vi "cRIO Main.vi"() -> ()   [LabVIEW 2013]
doc: "This example runs a background service that initializes and interacts with the Tag Bus Data framework. The service is designed to run continuously so that the framework can be reinitialized with a new configuration without rebooting the target. This can save time when iterating on a configuration.\n\nThe example includes a collection of VIs for sending and receiving messages from the engine service."
uses:
  TBD Message Service/SubVIs/command commands to rtexe process.ctl
  TBD Message Service/SubVIs/engine status data.ctl
  <vilib>/NI/Module Execution Interface/Engine Runtime/Execution States.ctl
  <vilib>/NI/Module Execution Interface/Engine Runtime/Fault.ctl
  <vilib>/NI/Tag Bus Module Framework/runtime/error classification.ctl
  TBD Message Service/SubVIs/queue name.ctl
  <vilib>/NI/Current Value Table/DataTypes/Double_Read.vi
  <vilib>/NI/Current Value Table/Type to Enum.vi
  <vilib>/NI/Current Value Table/DataTypes/Double_Type To Enum.vi
  <vilib>/NI/AMC/Read Termination Message.vi
  TBD Message Service/SubVIs/command to string.vi
  TBD Message Service/SubVIs/string to commands.vi
  <vilib>/NI/AMC/Create Single Message.vi
  <vilib>/NI/Current Value Table/FGVs/CVT Globals.vi
  <vilib>/NI/Current Value Table/FGVs/Tag Memory.vi
  <vilib>/NI/Current Value Table/Memory Block.vi
  <vilib>/NI/Current Value Table/DataTypes/Double_Memory Block.vi
  <vilib>/NI/AMC/Globals.vi
  TBD Message Service/TBD message service.lvlib
  <vilib>/NI/AMC/AMC.lvlib
  <vilib>/NI/Current Value Table/Current Value Table.lvlib
  <vilib>/NI/Module Execution Interface/Engine Runtime/Engine Runtime Interface.lvclass
  <vilib>/NI/Tag Bus Module Framework/runtime/TBM module execution interface.lvclass
panel:
  in  "Exit":bool
  in  "Reload":bool
  out "timed structures load":dbl
  out "CPU load average":dbl
  out "final error":errorcluster
  out "Lamp PWM":cluster{"Value":dbl, "Value":dbl}(graph)
  out "Temperature":cluster{"Value":dbl, "Value":dbl}(graph)
  out "system error":errorcluster
  out "engine statuses":T1[](array[typedef])
  out "command error":errorcluster
  out "commands":T5
  out "engine loaded":string
  out "load error":errorcluster
  out "Invalid Message":string
  in  "config. file path":path=path "/home/lvuser/natinst/bin/FullSystem.pcfg"
  # "Status Information"
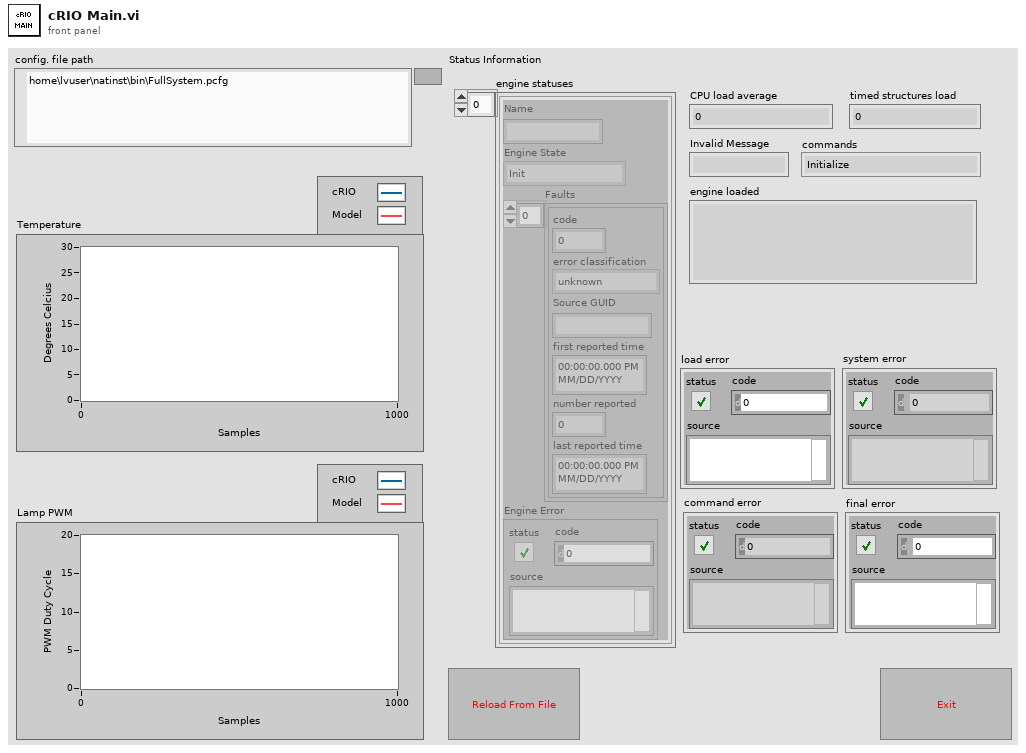
[diagram p1: front panel]
types:
  T1 = typedef "TBD message service.lvlib/engine status data.ctl" = cluster{"Name":string, "Engine State":T2, "Faults":T3[], "Engine Error":errorcluster}
  T2 = typedef "Engine Runtime Interface.lvclass/Execution States.ctl" = enum16{"Init", "Pre-Operational", "Safe-Operational", "Operational", "Stopped"}
  T3 = typedef "Engine Runtime Interface.lvclass/Fault.ctl" = cluster{"code":i32, "error classification":T4, "Source GUID":string, "first reported time":timestamp, "number reported":u32, "last reported time":timestamp}
  T4 = typedef "TBM module execution interface.lvclass/error classification.ctl" = enum16{"unknown", "none", "trivial", "recoverable", "critical"}
  T5 = typedef "TBD message service.lvlib/command commands to rtexe process.ctl" = enum16{"Initialize", "Add Search Paths", "Load from File", "Unload File", "Open All Engines", "Open Single Engine", "Initialize All Engines", "Initialize Single Engine", "Start All", "Start Single", "Pause All", "Pause Single", "Stop All", "Stop Single", "Close All", "Close Single", "Set Safe State All", "Set Safe State Single", "Get Status", "Exit", "Error", "Load Bitfile", "Unload Bitfile", "Clear Faults Single", "Clear Faults All"}
  T6 = typedef "TBD message service.lvlib/queue name.ctl" = enum16{"TOrtmainexec", "FROMrtmainexec"}
  T7 = typedef "AMC.lvlib/Message Queue.ctl" = refnum<queue>
  T8 = typedef "TBD message service.lvlib/common reponses to network process.ctl" = enum16{"System Error", "Load Report", "Action Response", "Engine Status"}
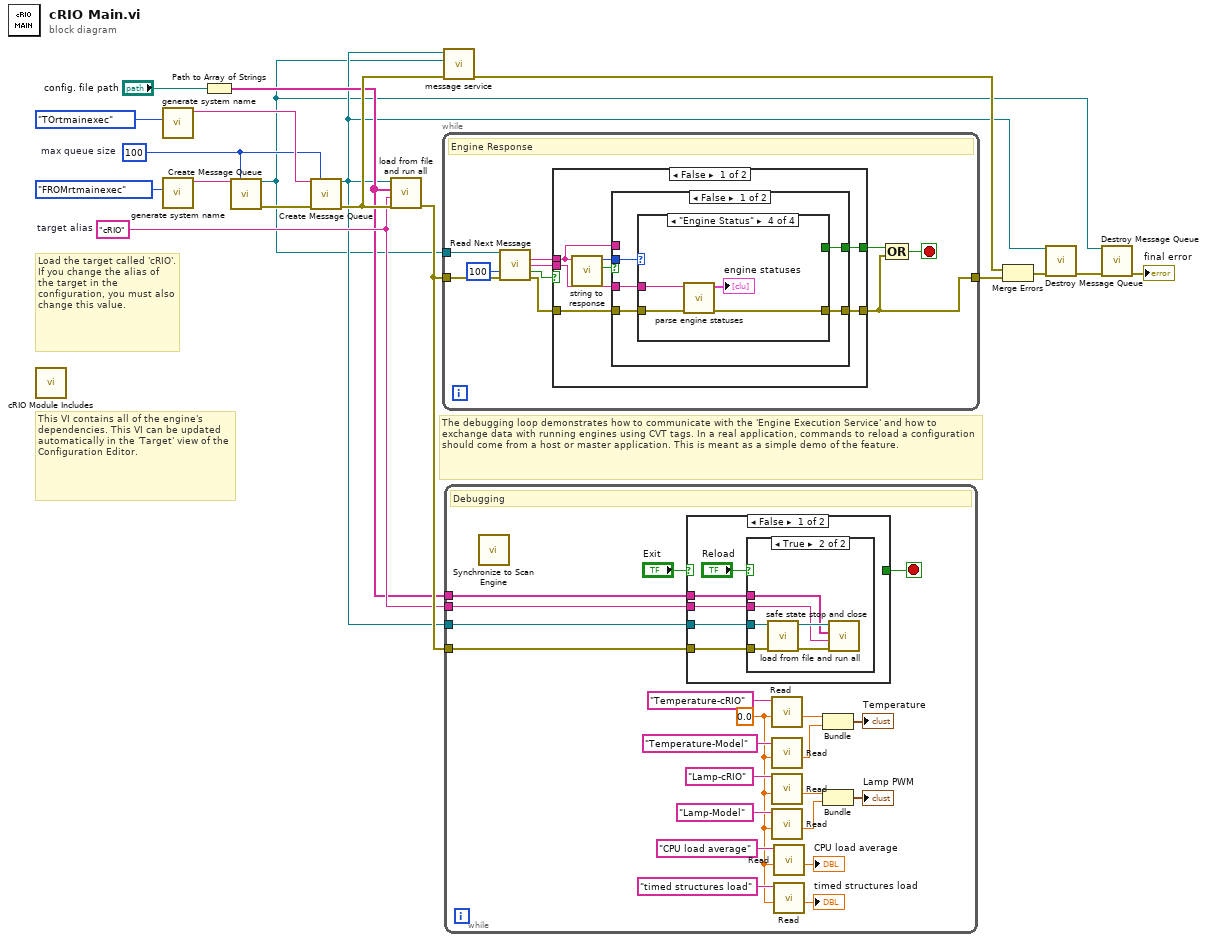
[diagram p0: block diagram]
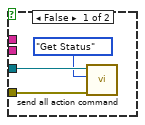
[diagram p2: hidden frame]
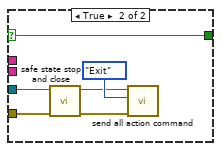
[diagram p3: hidden frame]
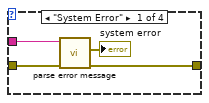
[diagram p4: hidden frame]
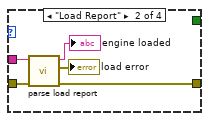
[diagram p5: hidden frame]
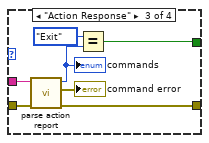
[diagram p6: hidden frame]
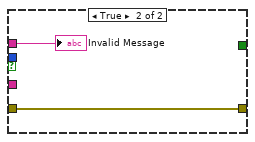
[diagram p7: hidden frame]
diagram:
  w12 = 100  # max queue size
  w9 = "cRIO"  # target alias
  # "This VI contains all of the engine's dependencies. This VI can be updated automatically in the 'Target' view of the Configuration Editor."
  # "Load the target called 'cRIO'. If you change the alias of the target in the configuration, you must also change this value."
  # "The debugging loop demonstrates how to communicate with the 'Engine Execution Service' and how to exchange data with running engines using CVT tags. In a real application, commands to reload a configuration should come from a host or master application. This is meant as a simple demo of the feature."
  n1 = call "cRIO Module Includes.vi"() -> ()  [unwired: 12 in]
  n2 = call "generate system name.vi"("queue type"=queue_name."TOrtmainexec" ("queue")) -> ("queue name"=w16:string)  [unwired: 10 in]
  n3 = call "generate system name.vi"("queue type"=queue_name."FROMrtmainexec" ("queue")) -> ("queue name"=w18:string)  [unwired: 10 in]
  n4 = Path to Array of Strings(0:"config. file path") -> (2:w8:string[])  [unwired: 1 out]
  n5 = call <vilib>:"Create Message Queue.vi"("message queue name"=w18, "max queue size (-1, unlimited)"=w12) -> ("message queue out"=w1:T7, "error out"=w17:errorcluster)  [unwired: 12 in]
  n6 = call <vilib>:"Create Message Queue.vi"("message queue name"=w16, "max queue size (-1, unlimited)"=w12, "error in"=w17) -> ("message queue out"=w2:T7, "error out"=w11:errorcluster)  [unwired: 11 in]
  n7 = call "load from file and run all.vi"("error in"=w11, "target alias"=w9, "tokenized path"=w8, "message queue in"=w2) -> ("error out"=w10:errorcluster)  [unwired: 6 in, 1 out]
  n8 = while {
    tunnel: w1 -> [w27]
    tunnel: w10 -> [w24]
    tunnel: [w19] -> w7
    stop <- w21 stop-if-true
    # "Engine Response"
    n9 = call <vilib>:"Read Next Message.vi"("message queue in"=w27, "timeout (1 ms)"=100, "error in"=w24) -> ("message name"=w26:string, "message value"=w20:string, "timed out?"=w23:bool, "error out"=w25:errorcluster)  [unwired: 5 in, 4 out]
    n10 = case shown="False" w23 {
      tunnel: w26 -> [w29 _]
      tunnel: [w34 _] -> w22
      tunnel: w25 -> [w32 w63]
      tunnel: [w31 w63] -> w19
      tunnel: w20 -> [w30 _]
      frame False {
        n11 = call "string to response.vi"("command string"=w29) -> ("invalid"=w35:bool, "responses"=w33:T8)  [unwired: 9 in]
        n12 = case shown="False" w35 {
          tunnel: w30 -> [w39 _]
          tunnel: [w36 _] -> w34
          tunnel: w33 -> [w40 _]
          tunnel: w32 -> [w38 w62]
          tunnel: [w37 w62] -> w31
          tunnel: w29 -> [_ w61]
          frame False {
            n13 = case shown="\"Engine Status\"" w40 {
              tunnel: w39 -> [w44 w49 w56 w60]
              tunnel: w38 -> [w43 w48 w55 w59]
              tunnel: [w41 w45 w53 w58] -> w37
              tunnel: [_ _ w50 _] -> w36
              frame "System Error" {
                n14 = call "parse error message.vi"("error in"=w43, "message data"=w44) -> ("error out"=w41:errorcluster, "system error"=→"system error":errorcluster)  [unwired: 8 in]
              }
              frame "Load Report" {
                n15 = call "parse load report.vi"("error in"=w48, "message data"=w49) -> ("error out"=w45:errorcluster, "load error"=→"load error":errorcluster, "engine loaded"=→"engine loaded":string)  [unwired: 7 in]
              }
              frame "Action Response" {
                n16 = call "parse action report.vi"("error in"=w55, "message data"=w56) -> ("error out"=w53:errorcluster, "command error"=→"command error":errorcluster, "commands"=w52:T5)  [unwired: 7 in]
                "commands" <- w52
                n17 = Equal?(x=command_commands_to_rtexe_process."Exit", y=w52) -> (x = y?=w50:bool)
              }
              frame "Engine Status" {
                n18 = call "parse engine statuses.vi"("error in"=w59, "message data"=w60) -> ("error out"=w58:errorcluster, "engine statuses"=→"engine statuses":T1[])  [unwired: 8 in]
              }
            }
          }
          frame True {
            "Invalid Message" <- w61
          }
        }
      }
      frame True {
      }
    }
    n19 = Compound Arithmetic op=OR(w22, w19) -> (w21:bool)
  }
  n20 = call "message service.vi"("error in"=w11, "response queue"=w1, "command queue"=w2) -> ("error out"=w6:errorcluster)  [unwired: 8 in]
  n21 = while {
    tunnel: w10 -> [w67]
    tunnel: w2 -> [w68]
    tunnel: w8 -> [w66]
    tunnel: w9 -> [w65]
    stop <- w64 stop-if-true
    w72 = 0.0 ("Default")
    # "Debugging"
    n22 = call <vilib>:"Synchronize to Scan Engine.vi"() -> ()  [unwired: 10 in, 2 out]
    n23 = case shown="False" "Exit" {
      selector: "Exit" -> [_ w102]
      tunnel: w68 -> [w88 w104]
      tunnel: w67 -> [w87 w103]
      tunnel: w66 -> [w86 _]
      tunnel: w65 -> [w85 _]
      tunnel: [_ w102] -> w64
      frame False {
        n24 = case shown="True" "Reload" {
          tunnel: w88 -> [w92 w98]
          tunnel: w87 -> [w91 w97]
          tunnel: w86 -> [_ w94]
          tunnel: w85 -> [_ w93]
          frame False {
            n25 = call "send all action command.vi"("error in"=w91, "commands"=command_commands_to_rtexe_process."Get Status", "message queue in"=w92) -> ()  [unwired: 7 in, 2 out]
          }
          frame True {
            n26 = call "safe state stop and close.vi"("error in"=w97, "message queue in"=w98) -> ("error out"=w95:errorcluster, "message queue out"=w96:T7)  [unwired: 8 in]
            n27 = call "load from file and run all.vi"("error in"=w95, "target alias"=w93, "tokenized path"=w94, "message queue in"=w96) -> ()  [unwired: 6 in, 2 out]
          }
        }
      }
      frame True {
        n28 = call "safe state stop and close.vi"("error in"=w103, "message queue in"=w104) -> ("error out"=w99:errorcluster, "message queue out"=w100:T7)  [unwired: 8 in]
        n29 = call "send all action command.vi"("error in"=w99, "commands"=command_commands_to_rtexe_process."Exit", "message queue in"=w100) -> ()  [unwired: 7 in, 2 out]
      }
    }
    n30 = call-poly <vilib>:"Read.vi"("Default"=w72, "Tag Name"="Temperature-cRIO") -> ("Value"=w80:dbl)  [unwired: 8 in, 1 out]
    n31 = call-poly <vilib>:"Read.vi"("Default"=w72, "Tag Name"="Temperature-Model") -> ("Value"=w79:dbl)  [unwired: 8 in, 1 out]
    n32 = call-poly <vilib>:"Read.vi"("Default"=w72, "Tag Name"="Lamp-cRIO") -> ("Value"=w78:dbl)  [unwired: 8 in, 1 out]
    n33 = call-poly <vilib>:"Read.vi"("Default"=w72, "Tag Name"="Lamp-Model") -> ("Value"=w77:dbl)  [unwired: 8 in, 1 out]
    n34 = call-poly <vilib>:"Read.vi"("Default"=w72, "Tag Name"="CPU load average") -> ("Value"=→"CPU load average":dbl)  [unwired: 8 in, 1 out]
    n35 = call-poly <vilib>:"Read.vi"("Default"=w72, "Tag Name"="timed structures load") -> ("Value"=→"timed structures load":dbl)  [unwired: 8 in, 1 out]
    n36 = Bundle("Value"=w80, "Value"=w79) -> (→"Temperature":cluster{"Value":dbl, "Value":dbl})  [unwired: 1 in]
    n37 = Bundle("Value"=w78, "Value"=w77) -> (→"Lamp PWM":cluster{"Value":dbl, "Value":dbl})  [unwired: 1 in]
  }
  n38 = Merge Errors(w6, w7) -> (w3:errorcluster)
  n39 = call <vilib>:"Destroy Message Queue.vi"("message queue in"=w2, "error in"=w3) -> ("error out"=w5:errorcluster)  [unwired: 11 in, 2 out]
  n40 = call <vilib>:"Destroy Message Queue.vi"("message queue in"=w1, "error in"=w5) -> ("error out"=→"final error":errorcluster)  [unwired: 11 in, 2 out]
